vi "Read Debug Behavior.vi"(8 "error in (no error)":errorcluster, 11 "Attribute":refnum<class "Attribute.lvclass">) -> (0 "error out":errorcluster, 2 "Behavior":T1, 3 "Attribute.StartupBehavior out":refnum<class "Attribute.Debug.lvclass">)   [LabVIEW 2019, in "SMO Debug.lvlib" / "Attribute.Debug.lvclass"]
uses:
  Attribute.Debug.lvclass
  DebugBehavior.ctl
  <vilib>/JKI/JKI SMO/Support/Attribute/Attribute.lvclass
  Attribute.Debug.lvclass/Attribute.Debug.ctl
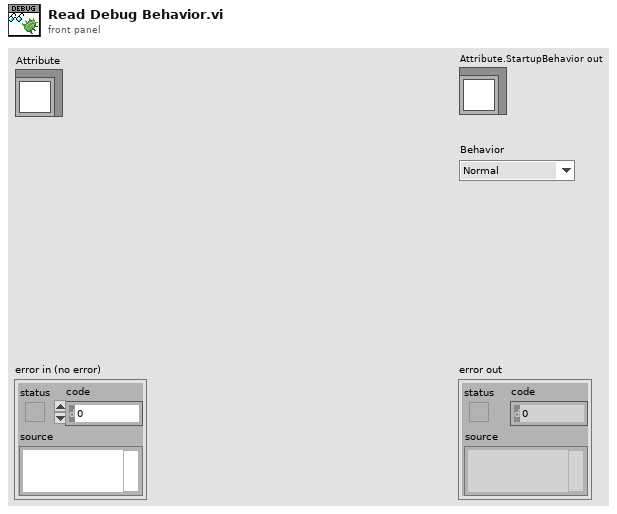
[diagram p1: front panel]
types:
  T1 = typedef "SMO Debug.lvlib/Attribute.Debug.lvclass/DebugBehavior.ctl" = enum16{"Normal", "Debug"}
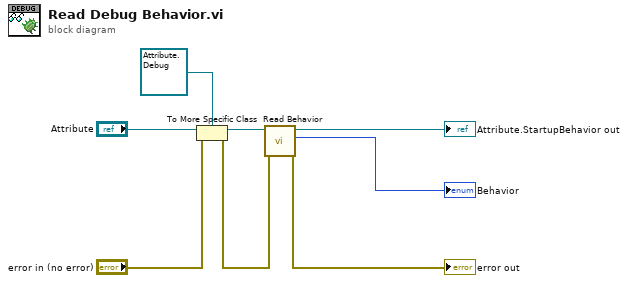
[diagram p0: block diagram]
diagram:
  n1 = To More Specific Class(target class=refnum<class "Attribute.Debug.lvclass"> refnum ("Attribute.StartupBehavior in"), reference="Attribute", error in="error in (no error)") -> (specific class reference=w6:refnum<class "Attribute.Debug.lvclass">, error out=w5:errorcluster)
  n2 = call "Read Behavior.vi"("error in (no error)"=w5, "Attribute.StartupBehavior in"=w6) -> ("error out"=→"error out":errorcluster, "Behavior"=→"Behavior":T1, "Attribute.StartupBehavior out"=→"Attribute.StartupBehavior out":refnum<class "Attribute.Debug.lvclass">)  [unwired: 7 in]
